vi "Configure Average Filter.vi"(0 "VISA resource name":refnum<visa-resource-name>, 1 "Count (10)":u32=10, 2 "Window (0)":dbl, 5 "Function (0: Voltage DC)":i32(ring) items=[" Voltage DC", "Voltage AC", "Current DC", "Current AC", "Resistance", "4-wire Resistance", "Diode", "Capacitance", "Temperature", "Continuity", "Frequency", "Period", "Voltage Ratio"], 7 "Enable Average Filter (F: Disable)":bool, 9 "Channel List (\"\")":string, 11 "error in (no error)":errorcluster, 12 "Average Filter Type (0: Repeat)":i32(ring) items=["Repeat", "Moving"]) -> (4 "VISA resource name out":refnum<visa-resource-name>, 15 "error out":errorcluster)   [LabVIEW 2024, in "Keithley DMM6500 DAQ6500 Series.lvlib"]
doc: "Configures average filter."
uses:
  Keithley DMM6500 DAQ6500 Series.lvlib
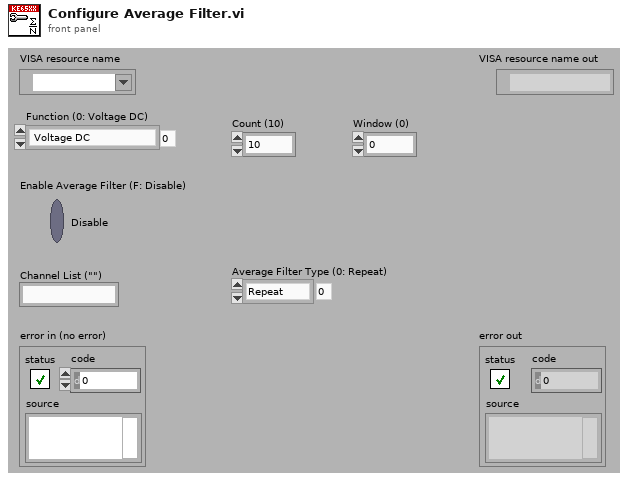
[diagram p1: front panel]
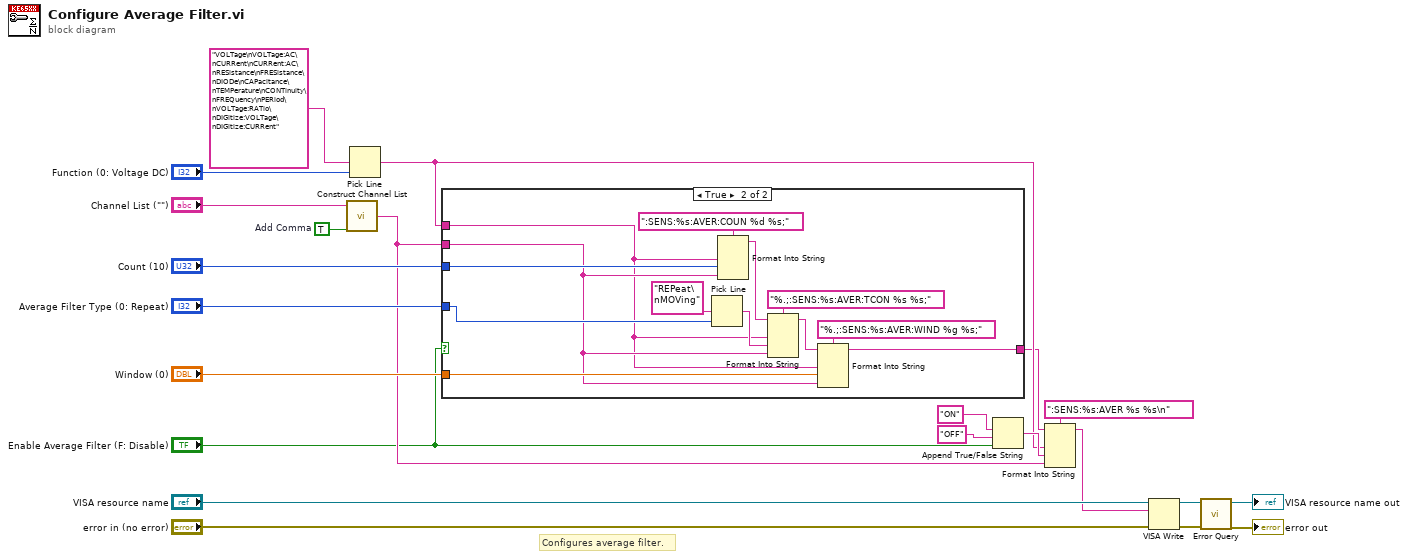
[diagram p0: block diagram]
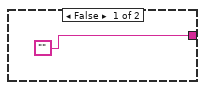
[diagram p2: hidden frame]
diagram:
  w12 = TRUE  # Add Comma
  # "Configures average filter."
  n1 = call "Construct Channel List.vi"("Add Comma (True)"=w12, "Channel List"="Channel List (\"\")") -> ("Channel List String"=w6:string)  [unwired: 1 in]
  n2 = Pick Line(multi-line string="VOLTage\nVOLTage:AC\nCURRent\nCURRent:AC\nRESistance\nFRESistance\nDIODe\nCAPacitance\nTEMPerature\nCONTinuity\nFREQuency\nPERiod\nVOLTage:RATio\nDIGitize:VOLTage\nDIGitize:CURRent", line index="Function (0: Voltage DC)") -> (output string=w5:string)  [unwired: 1 in]
  n3 = case shown="True" "Enable Average Filter (F: Disable)" {
    tunnel: "Count (10)" -> [_ w36]
    tunnel: "Window (0)" -> [_ w31]
    tunnel: "Average Filter Type (0: Repeat)" -> [_ w30]
    tunnel: w6 -> [_ w27]
    tunnel: w5 -> [_ w25]
    tunnel: ["" w24] -> w2
    frame False {
    }
    frame True {
      n4 = Pick Line(multi-line string="REPeat\nMOVing", line index=w30) -> (output string=w26:string)  [unwired: 1 in]
      n5 = Format Into String(format string=":SENS:%s:AVER:COUN %d %s;", w25, w36, w27) -> (resulting string=w35:string)  [unwired: 2 in, 1 out]
      n6 = Format Into String(format string="%.;:SENS:%s:AVER:TCON %s %s;", initial string=w35, w25, w26, w27) -> (resulting string=w33:string)  [unwired: 1 in, 1 out]
      n7 = Format Into String(format string="%.;:SENS:%s:AVER:WIND %g %s;", initial string=w33, w25, w31, w27) -> (resulting string=w24:string)  [unwired: 1 in, 1 out]
    }
  }
  n8 = Append True/False String(1:"Enable Average Filter (F: Disable)", 2:"OFF", 3:"ON") -> (0:w7:string)  [unwired: 1 in]
  n9 = Format Into String(format string=":SENS:%s:AVER %s %s\n", initial string=w2, w5, w7, w6) -> (resulting string=w3:string)  [unwired: 1 in, 1 out]
  n10 = VISA Write(VISA resource name="VISA resource name", write buffer=w3, error in (no error)="error in (no error)") -> (VISA resource name out=w18:refnum<visa-resource-name>, error out=w17:errorcluster)  [unwired: 1 out]
  n11 = call "Error Query.vi"("error in (no error)"=w17, "VISA resource name"=w18) -> ("error out"=→"error out":errorcluster, "VISA resource name out"=→"VISA resource name out":refnum<visa-resource-name>)  [unwired: 6 in, 2 out]
